vi "Reset.vi"(8 "error in (no error)":errorcluster, 11 "Multicolumn List Box View Model in":refnum<class "Multicolumn List Box View Model.lvclass">) -> (0 "error out":errorcluster, 3 "Multicolumn List Box View Model out":refnum<class "Multicolumn List Box View Model.lvclass">)   [LabVIEW 2020, in "Multicolumn List Box View Model.lvclass"]
uses:
  Multicolumn List Box View Model.lvclass
  Multicolumn List Box View Model.lvclass/Multicolumn List Box View Model.ctl
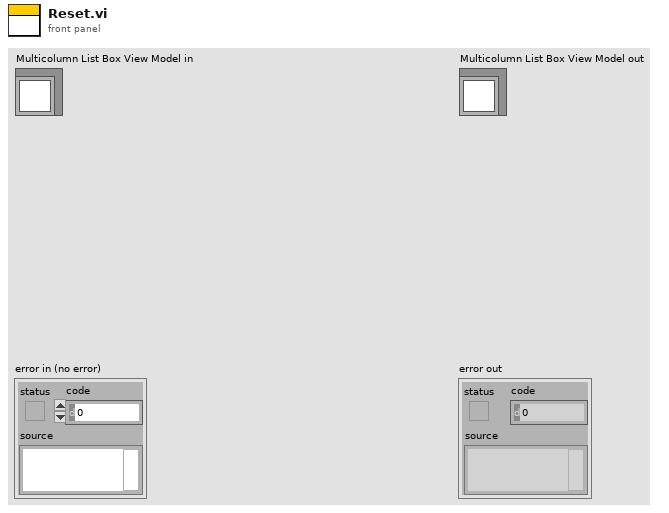
[diagram p1: front panel]
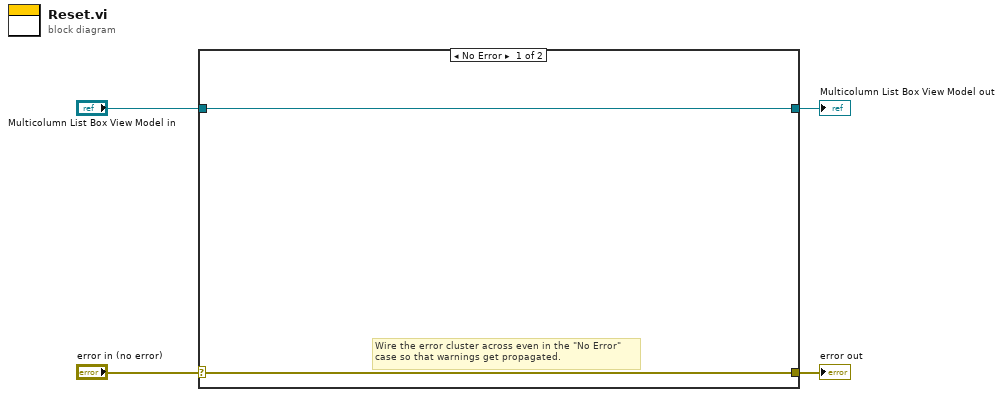
[diagram p0: block diagram]
diagram:
  n1 = case shown="No Error" "error in (no error)" {
    selector: "error in (no error)" -> [w5 w8]
    tunnel: [w5 w8] -> w3
    tunnel: [w6 w7] -> w1
    tunnel: "Multicolumn List Box View Model in" -> [w6 w7]
    frame No Error {
      # "Wire the error cluster across even in the \"No Error\"\ncase so that warnings get propagated."
    }
    frame Error {
    }
  }
  "error out" <- w3
  "Multicolumn List Box View Model out" <- w1
